vi "SRS_gate_time.vi"(8 "error in":errorcluster, 10 "Gate time":u16(ring) items=["0.1 seconds", "1.0 seconds", "10.0 seconds"], 11 "VISA in":refnum<visa-resource-name>="GPIB0::3::INSTR") -> (0 "error out":errorcluster, 3 "VISA out":refnum<visa-resource-name>)   [LabVIEW 2014]
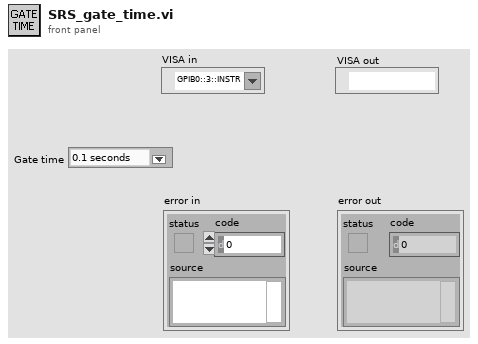
[diagram p1: front panel]
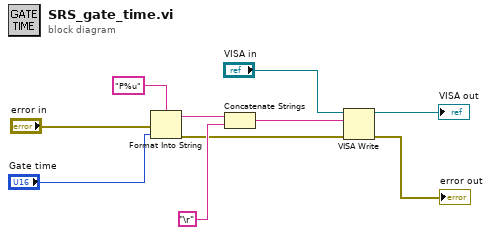
[diagram p0: block diagram]
diagram:
  n1 = Format Into String(format string="P%u", error in="error in", "Gate time") -> (resulting string=w2:string, error out=w3:errorcluster)  [unwired: 1 in]
  n2 = Concatenate Strings(w2, "\r") -> (w6:string)
  n3 = VISA Write(VISA resource name="VISA in", write buffer=w6, error in (no error)=w3) -> (VISA resource name out=→"VISA out":refnum<visa-resource-name>, error out=→"error out":errorcluster)  [unwired: 1 out]
